vi "Read data manual.vi"() -> ()   [LabVIEW 2018]
uses:
  Controls/READ CAN CLUSTER.ctl
  Controls/CLUSTER.ctl
  CAN/Tacho/Conf/FGV States.ctl
  CAN/CAN Write Data/Application/Common VIs/Read File Data.ctl
  Controls/READ CAN DATA.ctl
  f1f4e13e-2694-4935-9f44-7f0de9cfde9a.vi
  56b8a145-6b6a-4ebf-8834-6d6c23b684ec.vi
panel:
  in  "Write":bool
  in  "WRITE DATA":T1[](array[typedef])
  in  "START WRITING":bool
  out "MESSAGES":string
  out "READ DATA":T1[](array[typedef])
  in  "stop":bool
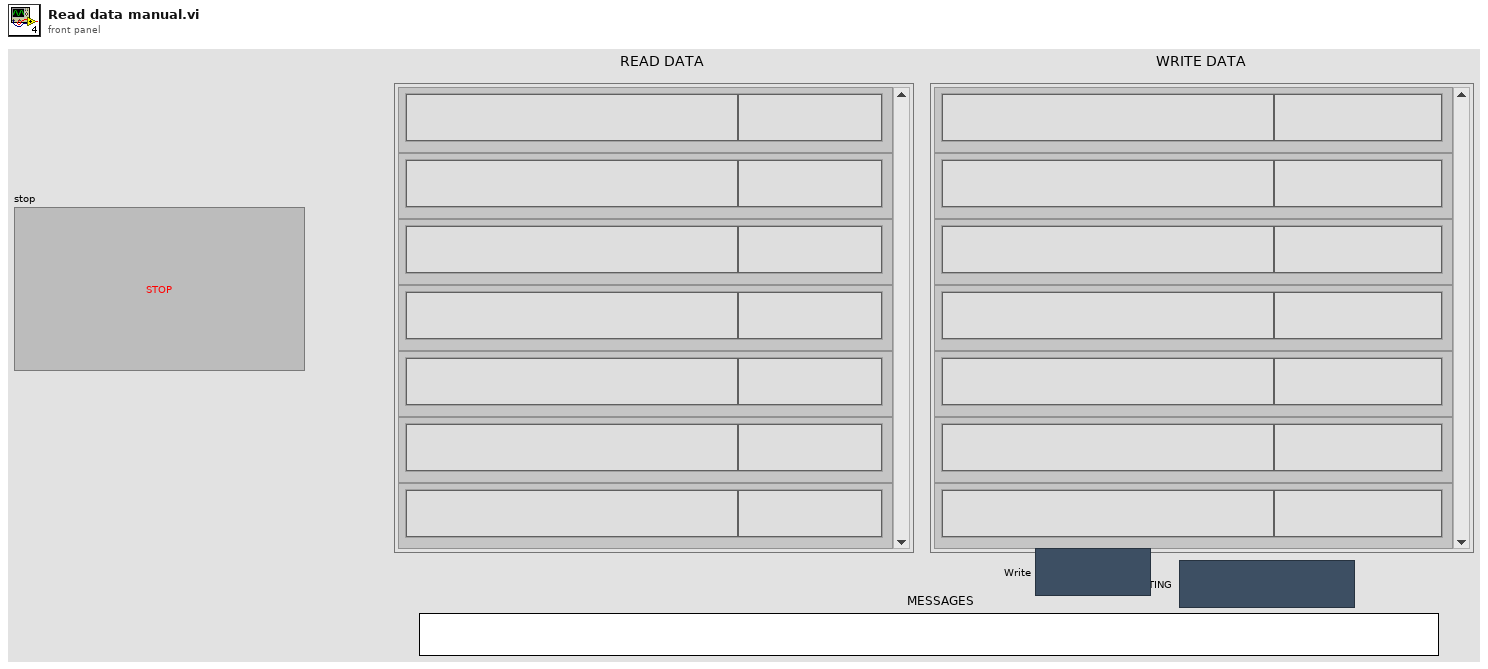
[diagram p1: front panel]
types:
  T1 = typedef "READ CAN CLUSTER.ctl" = cluster{"FUNCTION":string, "DATA":string}
  T2 = typedef "Read File Data.ctl" = enum16{"Get Data", "Set Data"}
  T3 = typedef "FGV States.ctl" = enum16{"OPEN", "READ", "CLOSE", "WRITE"}
  T4 = typedef "READ CAN DATA.ctl" = enum16{"SET", "GET"}
  T5 = typedef "CLUSTER.ctl" = cluster{"FUNCTION":string, "READ":bool, "WRITE":bool}
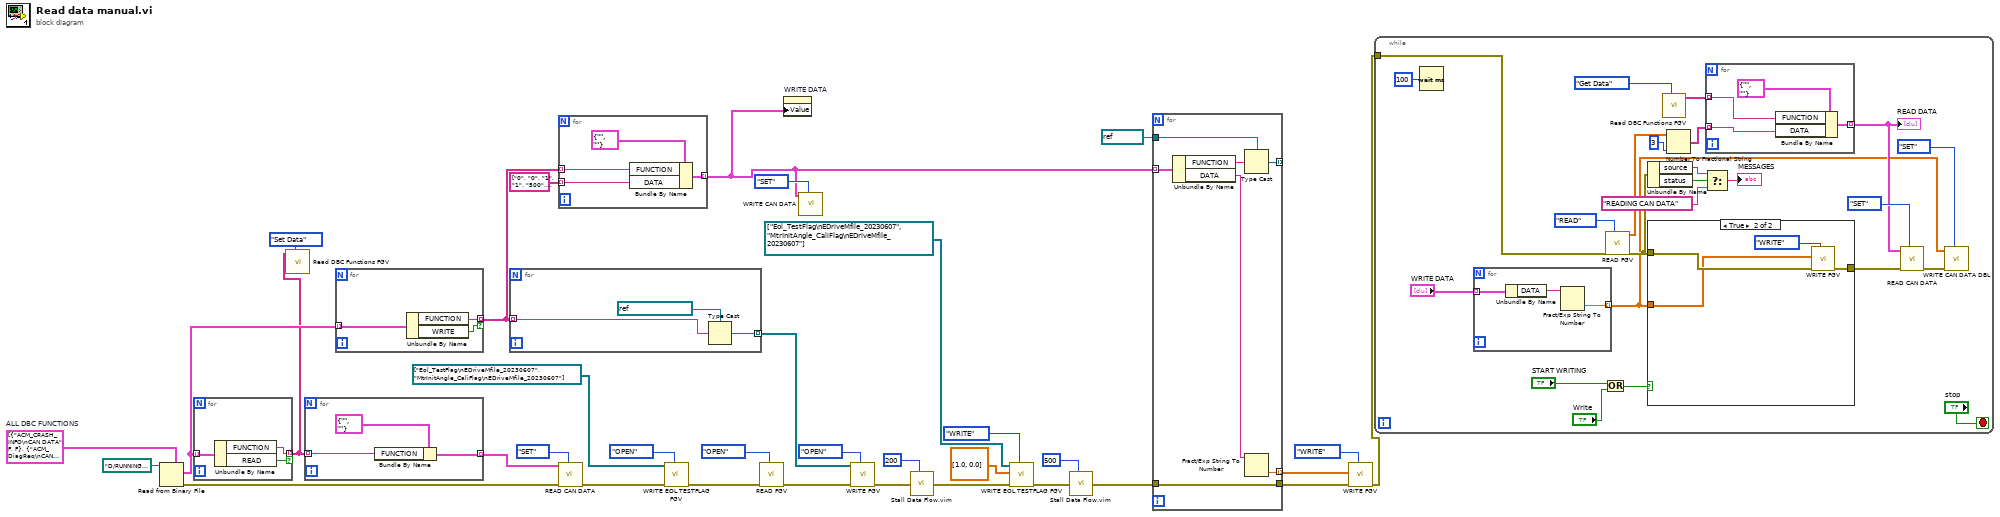
[diagram p0: block diagram]
diagram:
  w34 = T5[] [{"FUNCTION"="ACM_CRASH_INFO\nCAN DATA", "READ"=FALSE, "WRITE"=FALSE}, {"FUNCTION"="ACM_DiagReq\nCAN DATA", "READ"=FALSE, "WRITE"=FALSE}, {"FUNCTION"="ACM_DiagResp\nCAN DATA", "READ"=FALSE, "WRITE"=FALSE}, {"FUNCTION"="ACM_OCCUPANT_STATUS\nCAN DATA", "READ"=FALSE, "WRITE"=FALSE}, {"FUNCTION"="ACM_WarnMsg\nCAN DATA", "READ"=FALSE, "WRITE"=FALSE}, {"FUNCTION"="ADAS_AEB\nCAN DATA", "READ"=FALSE, "WRITE"=FALSE}, {"FUNCTION"="ADAS_AHB_DOW\nCAN DATA", "READ"=FALSE, "WRITE"=FALSE}, {"FUNCTION"="ADAS_APA_SLOT1INFO1\nCAN DATA", "READ"=FALSE, "WRITE"=FALSE}, {"FUNCTION"="ADAS_APA_SLOT1INFO2\nCAN DATA", "READ"=FALSE, "WRITE"=FALSE}, {"FUNCTION"="ADAS_APA_SLOT1INFO3\nCAN DATA", "READ"=FALSE, "WRITE"=FALSE}, {"FUNCTION"="ADAS_APA_SLOT2INFO1\nCAN DATA", "READ"=FALSE, "WRITE"=FALSE}, {"FUNCTION"="ADAS_APA_SLOT2INFO2\nCAN DATA", "READ"=FALSE, "WRITE"=FALSE}, {"FUNCTION"="ADAS_APA_SLOT2INFO3\nCAN DATA", "READ"=FALSE, "WRITE"=FALSE}, {"FUNCTION"="ADAS_APA_SLOT3INFO1\nCAN DATA", "READ"=FALSE, "WRITE"=FALSE}, {"FUNCTION"="ADAS_APA_SLOT3INFO2\nCAN DATA", "READ"=FALSE, "WRITE"=FALSE}, {"FUNCTION"="ADAS_APA_SLOT3INFO3\nCAN DATA", "READ"=FALSE, "WRITE"=FALSE}, {"FUNCTION"="ADAS_APA_SLOT4INFO1\nCAN DATA", "READ"=FALSE, "WRITE"=FALSE}, {"FUNCTION"="ADAS_APA_SLOT4INFO2\nCAN DATA", "READ"=FALSE, "WRITE"=FALSE}, {"FUNCTION"="ADAS_APA_SLOT4INFO3\nCAN DATA", "READ"=FALSE, "WRITE"=FALSE}, {"FUNCTION"="ADAS_APA_SLOT5INFO1\nCAN DATA", "READ"=FALSE, "WRITE"=FALSE}, {"FUNCTION"="ADAS_APA_SLOT5INFO2\nCAN DATA", "READ"=FALSE, "WRITE"=FALSE}, {"FUNCTION"="ADAS_APA_SLOT5INFO3\nCAN DATA", "READ"=FALSE, "WRITE"=FALSE}, {"FUNCTION"="ADAS_APA_SLOT6INFO1\nCAN DATA", "READ"=FALSE, "WRITE"=FALSE}, {"FUNCTION"="ADAS_APA_SLOT6INFO2\nCAN DATA", "READ"=FALSE, "WRITE"=FALSE}, {"FUNCTION"="ADAS_APA_SLOT6INFO3\nCAN DATA", "READ"=FALSE, "WRITE"=FALSE}, {"FUNCTION"="ADAS_AVM_Sts\nCAN DATA", "READ"=FALSE, "WRITE"=FALSE}, {"FUNCTION"="ADAS_BSD\nCAN DATA", "READ"=FALSE, "WRITE"=FALSE}, {"FUNCTION"="ADAS_CMP_ACC\nCAN DATA", "READ"=FALSE, "WRITE"=FALSE}, {"FUNCTION"="ADAS_CMP_CHECK\nCAN DATA", "READ"=FALSE, "WRITE"=FALSE}, {"FUNCTION"="ADAS_CMP_MHU\nCAN DATA", "READ"=FALSE, "WRITE"=FALSE}, {"FUNCTION"="ADAS_DMS_STATUS\nCAN DATA", "READ"=FALSE, "WRITE"=FALSE}, {"FUNCTION"="ADAS_DiagReq\nCAN DATA", "READ"=FALSE, "WRITE"=FALSE}, {"FUNCTION"="ADAS_DiagResp\nCAN DATA", "READ"=FALSE, "WRITE"=FALSE}, {"FUNCTION"="ADAS_ELK\nCAN DATA", "READ"=FALSE, "WRITE"=FALSE}, {"FUNCTION"="ADAS_FCW_RCTA\nCAN DATA", "READ"=FALSE, "WRITE"=FALSE}, {"FUNCTION"="ADAS_Immo_MHU\nCAN DATA", "READ"=FALSE, "WRITE"=FALSE}, {"FUNCTION"="ADAS_LDW_LKA\nCAN DATA", "READ"=FALSE, "WRITE"=FALSE}, {"FUNCTION"="ADAS_NM\nCAN DATA", "READ"=FALSE, "WRITE"=FALSE}, {"FUNCTION"="ADAS_PA\nCAN DATA", "READ"=FALSE, "WRITE"=FALSE}, {"FUNCTION"="ADAS_RP_Sts\nCAN DATA", "READ"=FALSE, "WRITE"=FALSE}, {"FUNCTION"="ADAS_Speed_Display\nCAN DATA", "READ"=FALSE, "WRITE"=FALSE}, {"FUNCTION"="ADAS_TSR_STATUS\nCAN DATA", "READ"=FALSE, "WRITE"=FALSE}, {"FUNCTION"="ADAS_WarnMsg\nCAN DATA", "READ"=FALSE, "WRITE"=FALSE}, {"FUNCTION"="AMP_DiagReq\nCAN DATA", "READ"=FALSE, "WRITE"=FALSE}, {"FUNCTION"="AMP_DiagResp\nCAN DATA", "READ"=FALSE, "WRITE"=FALSE}, {"FUNCTION"="AMP_MHUEQType\nCAN DATA", "READ"=FALSE, "WRITE"=FALSE}, {"FUNCTION"="AMP_MHU_Ann1_ModeSET\nCAN DATA", "READ"=FALSE, "WRITE"=FALSE}, {"FUNCTION"="AMP_MHU_Ann1_PromptsSET\nCAN DATA", "READ"=FALSE, "WRITE"=FALSE}, {"FUNCTION"="AMP_MHU_Ann2_SpeakerSET\nCAN DATA", "READ"=FALSE, "WRITE"=FALSE}, {"FUNCTION"="AMP_MHU_SET\nCAN DATA", "READ"=FALSE, "WRITE"=FALSE}, {"FUNCTION"="AMP_NM\nCAN DATA", "READ"=FALSE, "WRITE"=FALSE}, {"FUNCTION"="AMP_rDiagReq\nCAN DATA", "READ"=FALSE, "WRITE"=FALSE}, {"FUNCTION"="AMP_rDiagResp\nCAN DATA", "READ"=FALSE, "WRITE"=FALSE}, {"FUNCTION"="APA_FEEDBACK_MHU\nCAN DATA", "READ"=FALSE, "WRITE"=FALSE}, {"FUNCTION"="APA_SENSOR\nCAN DATA", "READ"=FALSE, "WRITE"=FALSE}, {"FUNCTION"="APM_DiagReq\nCAN DATA", "READ"=FALSE, "WRITE"=FALSE}, {"FUNCTION"="APM_DiagResp\nCAN DATA", "READ"=FALSE, "WRITE"=FALSE}, {"FUNCTION"="APM_WINDOW_POS\nCAN DATA", "READ"=FALSE, "WRITE"=FALSE}, {"FUNCTION"="APM_WarnMsg\nCAN DATA", "READ"=FALSE, "WRITE"=FALSE}, {"FUNCTION"="ASU_DiagReq\nCAN DATA", "READ"=FALSE, "WRITE"=FALSE}, {"FUNCTION"="ASU_DiagResp\nCAN DATA", "READ"=FALSE, "WRITE"=FALSE}, {"FUNCTION"="AVAS_DiagReq\nCAN DATA", "READ"=FALSE, "WRITE"=FALSE}, {"FUNCTION"="AVAS_DiagResp\nCAN DATA", "READ"=FALSE, "WRITE"=FALSE}, {"FUNCTION"="AVAS_STATUS\nCAN DATA", "READ"=FALSE, "WRITE"=FALSE}, {"FUNCTION"="BCM_ALM_warning\nCAN DATA", "READ"=FALSE, "WRITE"=FALSE}, {"FUNCTION"="BCM_BPM_DiagReq\nCAN DATA", "READ"=FALSE, "WRITE"=FALSE}, {"FUNCTION"="BCM_BPM_DiagResp\nCAN DATA", "READ"=FALSE, "WRITE"=FALSE}, {"FUNCTION"="BCM_CLAMP_STAT\nCAN DATA", "READ"=FALSE, "WRITE"=FALSE}, {"FUNCTION"="BCM_Comfort_Confirm_sts\nCAN DATA", "READ"=FALSE, "WRITE"=FALSE}, {"FUNCTION"="BCM_DiagReq\nCAN DATA", "READ"=FALSE, "WRITE"=FALSE}, {"FUNCTION"="BCM_DiagResp\nCAN DATA", "READ"=FALSE, "WRITE"=FALSE}, {"FUNCTION"="BCM_ENERGY_MANAGEMENT\nCAN DATA", "READ"=FALSE, "WRITE"=FALSE}, {"FUNCTION"="BCM_ENTRY_CONTROL\nCAN DATA", "READ"=FALSE, "WRITE"=FALSE}, {"FUNCTION"="BCM_FKS_STATUS\nCAN DATA", "READ"=FALSE, "WRITE"=FALSE}, {"FUNCTION"="BCM_LIGHT\nCAN DATA", "READ"=FALSE, "WRITE"=FALSE}, {"FUNCTION"="BCM_LOGICAL_CLAMP\nCAN DATA", "READ"=FALSE, "WRITE"=FALSE}, {"FUNCTION"="BCM_Mirror_Confirm_sts\nCAN DATA", "READ"=FALSE, "WRITE"=FALSE}, {"FUNCTION"="BCM_ODO\nCAN DATA", "READ"=FALSE, "WRITE"=FALSE}, {"FUNCTION"="BCM_RainLightSnr\nCAN DATA", "READ"=FALSE, "WRITE"=FALSE}, {"FUNCTION"="BCM_SCM_LIN_Info\nCAN DATA", "READ"=FALSE, "WRITE"=FALSE}, {"FUNCTION"="BCM_STAT_CENTRAL_LOCK\nCAN DATA", "READ"=FALSE, "WRITE"=FALSE}, {"FUNCTION"="BCM_STAT_DOOR_FLAP\nCAN DATA", "READ"=FALSE, "WRITE"=FALSE}, {"FUNCTION"="BCM_SunroofSts\nCAN DATA", "READ"=FALSE, "WRITE"=FALSE}, {"FUNCTION"="BCM_SunshadeSts\nCAN DATA", "READ"=FALSE, "WRITE"=FALSE}, {"FUNCTION"="BCM_SwitchSts\nCAN DATA", "READ"=FALSE, "WRITE"=FALSE}, {"FUNCTION"="BCM_TERMINAL\nCAN DATA", "READ"=FALSE, "WRITE"=FALSE}, {"FUNCTION"="BCM_VEHICLE_IDENT_NUMBER\nCAN DATA", "READ"=FALSE, "WRITE"=FALSE}, {"FUNCTION"="BCM_VOLTAGE\nCAN DATA", "READ"=FALSE, "WRITE"=FALSE}, {"FUNCTION"="BCM_WarnMsg\nCAN DATA", "READ"=FALSE, "WRITE"=FALSE}, {"FUNCTION"="BMS_CellTemp\nCAN DATA", "READ"=FALSE, "WRITE"=FALSE}, {"FUNCTION"="BMS_ChgParamReq\nCAN DATA", "READ"=FALSE, "WRITE"=FALSE}, {"FUNCTION"="BMS_CurMeas\nCAN DATA", "READ"=FALSE, "WRITE"=FALSE}, {"FUNCTION"="BMS_DiagReq\nCAN DATA", "READ"=FALSE, "WRITE"=FALSE}, {"FUNCTION"="BMS_DiagResp\nCAN DATA", "READ"=FALSE, "WRITE"=FALSE}, {"FUNCTION"="BMS_HVMeas1\nCAN DATA", "READ"=FALSE, "WRITE"=FALSE}, {"FUNCTION"="BMS_Sts\nCAN DATA", "READ"=FALSE, "WRITE"=FALSE}, {"FUNCTION"="BMS_WarnMsg\nCAN DATA", "READ"=FALSE, "WRITE"=FALSE}, {"FUNCTION"="CCUF_DiagReq\nCAN DATA", "READ"=FALSE, "WRITE"=FALSE}, {"FUNCTION"="CCUF_DiagResp\nCAN DATA", "READ"=FALSE, "WRITE"=FALSE}, {"FUNCTION"="CCUR_DiagReq\nCAN DATA", "READ"=FALSE, "WRITE"=FALSE}, {"FUNCTION"="CCUR_DiagResp\nCAN DATA", "READ"=FALSE, "WRITE"=FALSE}, {"FUNCTION"="CCU_STATUS\nCAN DATA", "READ"=FALSE, "WRITE"=FALSE}, {"FUNCTION"="CCU_TEMP_PRESSURE\nCAN DATA", "READ"=FALSE, "WRITE"=FALSE}, {"FUNCTION"="CCU_WarnMsg\nCAN DATA", "READ"=FALSE, "WRITE"=FALSE}, {"FUNCTION"="CPD_DiagReq\nCAN DATA", "READ"=FALSE, "WRITE"=FALSE}, {"FUNCTION"="CPD_DiagResp\nCAN DATA", "READ"=FALSE, "WRITE"=FALSE}, {"FUNCTION"="CPD_NM\nCAN DATA", "READ"=FALSE, "WRITE"=FALSE}, {"FUNCTION"="CPD_OUTPUT\nCAN DATA", "READ"=FALSE, "WRITE"=FALSE}, {"FUNCTION"="CPD_WarnMsg\nCAN DATA", "READ"=FALSE, "WRITE"=FALSE}, {"FUNCTION"="CPD_rDiagReq\nCAN DATA", "READ"=FALSE, "WRITE"=FALSE}, {"FUNCTION"="CPD_rDiagResp\nCAN DATA", "READ"=FALSE, "WRITE"=FALSE}, {"FUNCTION"="Camera_Lane\nCAN DATA", "READ"=FALSE, "WRITE"=FALSE}, {"FUNCTION"="Camera_Object01\nCAN DATA", "READ"=FALSE, "WRITE"=FALSE}, {"FUNCTION"="Camera_Object02\nCAN DATA", "READ"=FALSE, "WRITE"=FALSE}, {"FUNCTION"="Camera_Object03\nCAN DATA", "READ"=FALSE, "WRITE"=FALSE}, {"FUNCTION"="Camera_Object04\nCAN DATA", "READ"=FALSE, "WRITE"=FALSE}, {"FUNCTION"="Camera_Object05\nCAN DATA", "READ"=FALSE, "WRITE"=FALSE}, {"FUNCTION"="Camera_Object06\nCAN DATA", "READ"=FALSE, "WRITE"=FALSE}, {"FUNCTION"="Camera_leftlane\nCAN DATA", "READ"=FALSE, "WRITE"=FALSE}, {"FUNCTION"="Camera_rightlane\nCAN DATA", "READ"=FALSE, "WRITE"=FALSE}, {"FUNCTION"="DCM_APM_DiagReq\nCAN DATA", "READ"=FALSE, "WRITE"=FALSE}, {"FUNCTION"="DCM_APM_DiagResp\nCAN DATA", "READ"=FALSE, "WRITE"=FALSE}, {"FUNCTION"="DIAG_Req_All_CAN\nCAN DATA", "READ"=FALSE, "WRITE"=FALSE}, {"FUNCTION"="DIAG_Req_All_Ecu\nCAN DATA", "READ"=FALSE, "WRITE"=FALSE}, {"FUNCTION"="DIAG_Req_Info\nCAN DATA", "READ"=FALSE, "WRITE"=FALSE}, {"FUNCTION"="DMS_Status\nCAN DATA", "READ"=FALSE, "WRITE"=FALSE}, {"FUNCTION"="Diag_Request_ECU\nCAN DATA", "READ"=FALSE, "WRITE"=FALSE}, {"FUNCTION"="EASC_Confirm_sts\nCAN DATA", "READ"=FALSE, "WRITE"=FALSE}, {"FUNCTION"="EASC_DiagReq\nCAN DATA", "READ"=FALSE, "WRITE"=FALSE}, {"FUNCTION"="EASC_DiagResp\nCAN DATA", "READ"=FALSE, "WRITE"=FALSE}, {"FUNCTION"="EASC_NM\nCAN DATA", "READ"=FALSE, "WRITE"=FALSE}, {"FUNCTION"="EASC_WarnMsg\nCAN DATA", "READ"=FALSE, "WRITE"=FALSE}, {"FUNCTION"="EASC_rDiagReq\nCAN DATA", "READ"=FALSE, "WRITE"=FALSE}, {"FUNCTION"="EASC_rDiagResp\nCAN DATA", "READ"=FALSE, "WRITE"=FALSE}, {"FUNCTION"="EDS_F_DiagReq\nCAN DATA", "READ"=FALSE, "WRITE"=FALSE}, {"FUNCTION"="EDS_F_DiagResp\nCAN DATA", "READ"=FALSE, "WRITE"=FALSE}, {"FUNCTION"="EDS_F_WarnMsg\nCAN DATA", "READ"=FALSE, "WRITE"=FALSE}, {"FUNCTION"="EDS_OutPut_FR\nCAN DATA", "READ"=FALSE, "WRITE"=FALSE}, {"FUNCTION"="EDS_OutPut_RR\nCAN DATA", "READ"=FALSE, "WRITE"=FALSE}, {"FUNCTION"="EDS_R_DiagReq\nCAN DATA", "READ"=FALSE, "WRITE"=FALSE}, {"FUNCTION"="EDS_R_DiagResp\nCAN DATA", "READ"=FALSE, "WRITE"=FALSE}, {"FUNCTION"="EDS_R_WarnMsg\nCAN DATA", "READ"=FALSE, "WRITE"=FALSE}, {"FUNCTION"="EPS2_DiagReq\nCAN DATA", "READ"=FALSE, "WRITE"=FALSE}, {"FUNCTION"="EPS2_DiagResp\nCAN DATA", "READ"=FALSE, "WRITE"=FALSE}, {"FUNCTION"="EPS_DiagReq\nCAN DATA", "READ"=FALSE, "WRITE"=FALSE}, {"FUNCTION"="EPS_DiagResp\nCAN DATA", "READ"=FALSE, "WRITE"=FALSE}, {"FUNCTION"="EPS_WarnMsg\nCAN DATA", "READ"=FALSE, "WRITE"=FALSE}, {"FUNCTION"="ETG_DiagReq\nCAN DATA", "READ"=FALSE, "WRITE"=FALSE}, {"FUNCTION"="ETG_DiagResp\nCAN DATA", "READ"=FALSE, "WRITE"=FALSE}, {"FUNCTION"="ETG_STATUS\nCAN DATA", "READ"=FALSE, "WRITE"=FALSE}, {"FUNCTION"="ETG_WarnMsg\nCAN DATA", "READ"=FALSE, "WRITE"=FALSE}, {"FUNCTION"="GS_DiagReq\nCAN DATA", "READ"=FALSE, "WRITE"=FALSE}, {"FUNCTION"="GS_DiagResp\nCAN DATA", "READ"=FALSE, "WRITE"=FALSE}, {"FUNCTION"="GS_WarnMsg\nCAN DATA", "READ"=FALSE, "WRITE"=FALSE}, {"FUNCTION"="GW_BCM_Immo_MHU_Byte\nCAN DATA", "READ"=FALSE, "WRITE"=FALSE}, {"FUNCTION"="GW_BCM_RemoteCtrlSts\nCAN DATA", "READ"=FALSE, "WRITE"=FALSE}, {"FUNCTION"="HOD_Heating\nCAN DATA", "READ"=FALSE, "WRITE"=FALSE}, {"FUNCTION"="HOD_Heating_FDBK\nCAN DATA", "READ"=FALSE, "WRITE"=FALSE}, {"FUNCTION"="HUD_DiagReq\nCAN DATA", "READ"=FALSE, "WRITE"=FALSE}, {"FUNCTION"="HUD_DiagResp\nCAN DATA", "READ"=FALSE, "WRITE"=FALSE}, {"FUNCTION"="HUD_ECU_Status\nCAN DATA", "READ"=FALSE, "WRITE"=FALSE}, {"FUNCTION"="HUD_NM\nCAN DATA", "READ"=FALSE, "WRITE"=FALSE}, {"FUNCTION"="HUD_State\nCAN DATA", "READ"=FALSE, "WRITE"=FALSE}, {"FUNCTION"="HUD_WarnMsg\nCAN DATA", "READ"=FALSE, "WRITE"=FALSE}, {"FUNCTION"="HUD_rDiagReq\nCAN DATA", "READ"=FALSE, "WRITE"=FALSE}, {"FUNCTION"="HUD_rDiagResp\nCAN DATA", "READ"=FALSE, "WRITE"=FALSE}, {"FUNCTION"="IC_BORD_COMP_TRIP_A\nCAN DATA", "READ"=FALSE, "WRITE"=FALSE}, {"FUNCTION"="IC_BORD_COMP_TRIP_Auto\nCAN DATA", "READ"=FALSE, "WRITE"=FALSE}, {"FUNCTION"="IC_BORD_COMP_TRIP_B\nCAN DATA", "READ"=FALSE, "WRITE"=FALSE}, {"FUNCTION"="IC_MILEAGE\nCAN DATA", "READ"=FALSE, "WRITE"=FALSE}, {"FUNCTION"="IC_ODO\nCAN DATA", "READ"=FALSE, "WRITE"=FALSE}, {"FUNCTION"="IC_RELATIVIME\nCAN DATA", "READ"=FALSE, "WRITE"=FALSE}, {"FUNCTION"="IC_SENSOR\nCAN DATA", "READ"=FALSE, "WRITE"=FALSE}, {"FUNCTION"="IC_STAT_AIRBAG\nCAN DATA", "READ"=FALSE, "WRITE"=FALSE}, {"FUNCTION"="IDB_ACC_LONG_LAT_YAW\nCAN DATA", "READ"=FALSE, "WRITE"=FALSE}, {"FUNCTION"="IDB_DiagReq\nCAN DATA", "READ"=FALSE, "WRITE"=FALSE}, {"FUNCTION"="IDB_DiagResp\nCAN DATA", "READ"=FALSE, "WRITE"=FALSE}, {"FUNCTION"="IDB_EPB_STATUS\nCAN DATA", "READ"=FALSE, "WRITE"=FALSE}, {"FUNCTION"="IDB_FUNCTION\nCAN DATA", "READ"=FALSE, "WRITE"=FALSE}, {"FUNCTION"="IDB_MILEAGE\nCAN DATA", "READ"=FALSE, "WRITE"=FALSE}, {"FUNCTION"="IDB_STATUS\nCAN DATA", "READ"=FALSE, "WRITE"=FALSE}, {"FUNCTION"="IDB_V_VEH\nCAN DATA", "READ"=FALSE, "WRITE"=FALSE}, {"FUNCTION"="IDB_WarnMsg\nCAN DATA", "READ"=FALSE, "WRITE"=FALSE}, {"FUNCTION"="LDML_LIGHT\nCAN DATA", "READ"=FALSE, "WRITE"=FALSE}, {"FUNCTION"="LDMR_LIGHT\nCAN DATA", "READ"=FALSE, "WRITE"=FALSE}, {"FUNCTION"="LDM_L_DiagReq\nCAN DATA", "READ"=FALSE, "WRITE"=FALSE}, {"FUNCTION"="LDM_L_DiagResp\nCAN DATA", "READ"=FALSE, "WRITE"=FALSE}, {"FUNCTION"="LDM_R_DiagReq\nCAN DATA", "READ"=FALSE, "WRITE"=FALSE}, {"FUNCTION"="LDM_R_DiagResp\nCAN DATA", "READ"=FALSE, "WRITE"=FALSE}, {"FUNCTION"="MFS_Control_Button\nCAN DATA", "READ"=FALSE, "WRITE"=FALSE}, {"FUNCTION"="MHU_ADAS_RP_Ctrl\nCAN DATA", "READ"=FALSE, "WRITE"=FALSE}, {"FUNCTION"="MHU_ADAS_RSSI\nCAN DATA", "READ"=FALSE, "WRITE"=FALSE}, {"FUNCTION"="MHU_ADAS_req\nCAN DATA", "READ"=FALSE, "WRITE"=FALSE}, {"FUNCTION"="MHU_AMP_Ann1_ModeSET\nCAN DATA", "READ"=FALSE, "WRITE"=FALSE}, {"FUNCTION"="MHU_AMP_Ann1_PromptsSET\nCAN DATA", "READ"=FALSE, "WRITE"=FALSE}, {"FUNCTION"="MHU_AMP_Ann2_SpeakerSET\nCAN DATA", "READ"=FALSE, "WRITE"=FALSE}, {"FUNCTION"="MHU_AmpEQType\nCAN DATA", "READ"=FALSE, "WRITE"=FALSE}, {"FUNCTION"="MHU_AmpSET\nCAN DATA", "READ"=FALSE, "WRITE"=FALSE}, {"FUNCTION"="MHU_Auth_Immo\nCAN DATA", "READ"=FALSE, "WRITE"=FALSE}, {"FUNCTION"="MHU_Auth_Immo_ADAS\nCAN DATA", "READ"=FALSE, "WRITE"=FALSE}, {"FUNCTION"="MHU_Avas_Setting\nCAN DATA", "READ"=FALSE, "WRITE"=FALSE}, {"FUNCTION"="MHU_BCM_Color_Req\nCAN DATA", "READ"=FALSE, "WRITE"=FALSE}, {"FUNCTION"="MHU_BCM_DoorsCtrl\nCAN DATA", "READ"=FALSE, "WRITE"=FALSE}, {"FUNCTION"="MHU_BCM_HornLightControl\nCAN DATA", "READ"=FALSE, "WRITE"=FALSE}, {"FUNCTION"="MHU_BCM_IntensityTiming_Req\nCAN DATA", "READ"=FALSE, "WRITE"=FALSE}, {"FUNCTION"="MHU_BCM_RemoteClampCtrl\nCAN DATA", "READ"=FALSE, "WRITE"=FALSE}, {"FUNCTION"="MHU_CCUF_ClimateSetting\nCAN DATA", "READ"=FALSE, "WRITE"=FALSE}, {"FUNCTION"="MHU_CCUR_ClimateSetting\nCAN DATA", "READ"=FALSE, "WRITE"=FALSE}, {"FUNCTION"="MHU_CPD_Confirm\nCAN DATA", "READ"=FALSE, "WRITE"=FALSE}, {"FUNCTION"="MHU_CarMode_Switch\nCAN DATA", "READ"=FALSE, "WRITE"=FALSE}, {"FUNCTION"="MHU_ComfortSetting\nCAN DATA", "READ"=FALSE, "WRITE"=FALSE}, {"FUNCTION"="MHU_DATE_TIME\nCAN DATA", "READ"=FALSE, "WRITE"=FALSE}, {"FUNCTION"="MHU_DIGIT_SPEED\nCAN DATA", "READ"=FALSE, "WRITE"=FALSE}, {"FUNCTION"="MHU_DMS_STATUS\nCAN DATA", "READ"=FALSE, "WRITE"=FALSE}, {"FUNCTION"="MHU_DRIVER_INFO\nCAN DATA", "READ"=FALSE, "WRITE"=FALSE}, {"FUNCTION"="MHU_DiagReq\nCAN DATA", "READ"=FALSE, "WRITE"=FALSE}, {"FUNCTION"="MHU_DiagResp\nCAN DATA", "READ"=FALSE, "WRITE"=FALSE}, {"FUNCTION"="MHU_DoorSetting\nCAN DATA", "READ"=FALSE, "WRITE"=FALSE}, {"FUNCTION"="MHU_EvSetting\nCAN DATA", "READ"=FALSE, "WRITE"=FALSE}, {"FUNCTION"="MHU_FEEDBACK_APA\nCAN DATA", "READ"=FALSE, "WRITE"=FALSE}, {"FUNCTION"="MHU_FOTA_ReqAll\nCAN DATA", "READ"=FALSE, "WRITE"=FALSE}, {"FUNCTION"="MHU_FOTA_STATUS\nCAN DATA", "READ"=FALSE, "WRITE"=FALSE}, {"FUNCTION"="MHU_HEADLAMP_CTL\nCAN DATA", "READ"=FALSE, "WRITE"=FALSE}, {"FUNCTION"="MHU_HUD_BASE\nCAN DATA", "READ"=FALSE, "WRITE"=FALSE}, {"FUNCTION"="MHU_HUD_Info_1\nCAN DATA", "READ"=FALSE, "WRITE"=FALSE}, {"FUNCTION"="MHU_HUD_NAV_DISP\nCAN DATA", "READ"=FALSE, "WRITE"=FALSE}, {"FUNCTION"="MHU_HUD_NAV_GuidanceCont\nCAN DATA", "READ"=FALSE, "WRITE"=FALSE}, {"FUNCTION"="MHU_HudPositionSetting\nCAN DATA", "READ"=FALSE, "WRITE"=FALSE}, {"FUNCTION"="MHU_HudSetting\nCAN DATA", "READ"=FALSE, "WRITE"=FALSE}, {"FUNCTION"="MHU_IDB_Mode_Select\nCAN DATA", "READ"=FALSE, "WRITE"=FALSE}, {"FUNCTION"="MHU_ISA_Speed\nCAN DATA", "READ"=FALSE, "WRITE"=FALSE}, {"FUNCTION"="MHU_LightSetting\nCAN DATA", "READ"=FALSE, "WRITE"=FALSE}, {"FUNCTION"="MHU_MirrorAdjust\nCAN DATA", "READ"=FALSE, "WRITE"=FALSE}, {"FUNCTION"="MHU_NAV_JUNC_INFO\nCAN DATA", "READ"=FALSE, "WRITE"=FALSE}, {"FUNCTION"="MHU_NM\nCAN DATA", "READ"=FALSE, "WRITE"=FALSE}, {"FUNCTION"="MHU_SEAT_CONTROL\nCAN DATA", "READ"=FALSE, "WRITE"=FALSE}, {"FUNCTION"="MHU_STATUS\nCAN DATA", "READ"=FALSE, "WRITE"=FALSE}, {"FUNCTION"="MHU_SeatVentHeat\nCAN DATA", "READ"=FALSE, "WRITE"=FALSE}, {"FUNCTION"="MHU_SteeringAdjust\nCAN DATA", "READ"=FALSE, "WRITE"=FALSE}, {"FUNCTION"="MHU_UserProfile\nCAN DATA", "READ"=FALSE, "WRITE"=FALSE}, {"FUNCTION"="MHU_WindowSetting\nCAN DATA", "READ"=FALSE, "WRITE"=FALSE}, {"FUNCTION"="MRGEN_DiagReq\nCAN DATA", "READ"=FALSE, "WRITE"=FALSE}, {"FUNCTION"="MRGEN_DiagResp\nCAN DATA", "READ"=FALSE, "WRITE"=FALSE}, {"FUNCTION"="OCS_P_DiagReq\nCAN DATA", "READ"=FALSE, "WRITE"=FALSE}, {"FUNCTION"="OCS_P_DiagResp\nCAN DATA", "READ"=FALSE, "WRITE"=FALSE}, {"FUNCTION"="POD_DCDC_DiagReq\nCAN DATA", "READ"=FALSE, "WRITE"=FALSE}, {"FUNCTION"="POD_DCDC_DiagResp\nCAN DATA", "READ"=FALSE, "WRITE"=FALSE}, {"FUNCTION"="POD_GW_Request\nCAN DATA", "READ"=FALSE, "WRITE"=FALSE}, {"FUNCTION"="POD_GW_Response\nCAN DATA", "READ"=FALSE, "WRITE"=FALSE}, {"FUNCTION"="POD_OBC_DiagReq\nCAN DATA", "READ"=FALSE, "WRITE"=FALSE}, {"FUNCTION"="POD_OBC_DiagResp\nCAN DATA", "READ"=FALSE, "WRITE"=FALSE}, {"FUNCTION"="POD_WarnMsg\nCAN DATA", "READ"=FALSE, "WRITE"=FALSE}, {"FUNCTION"="PSM_D_DiagReq\nCAN DATA", "READ"=FALSE, "WRITE"=FALSE}, {"FUNCTION"="PSM_D_DiagResp\nCAN DATA", "READ"=FALSE, "WRITE"=FALSE}, {"FUNCTION"="PSM_D_SEAT_CONTROL\nCAN DATA", "READ"=FALSE, "WRITE"=FALSE}, {"FUNCTION"="PSM_SEAT_POSITION\nCAN DATA", "READ"=FALSE, "WRITE"=FALSE}, {"FUNCTION"="PSM_WarnMsg\nCAN DATA", "READ"=FALSE, "WRITE"=FALSE}, {"FUNCTION"="RCU_DiagReq\nCAN DATA", "READ"=FALSE, "WRITE"=FALSE}, {"FUNCTION"="RCU_DiagResp\nCAN DATA", "READ"=FALSE, "WRITE"=FALSE}, {"FUNCTION"="RCU_WarnMsg\nCAN DATA", "READ"=FALSE, "WRITE"=FALSE}, {"FUNCTION"="SAS_Sensor\nCAN DATA", "READ"=FALSE, "WRITE"=FALSE}, {"FUNCTION"="SCAM_DiagReq\nCAN DATA", "READ"=FALSE, "WRITE"=FALSE}, {"FUNCTION"="SCAM_DiagResp\nCAN DATA", "READ"=FALSE, "WRITE"=FALSE}, {"FUNCTION"="SCM_Raw_Status\nCAN DATA", "READ"=FALSE, "WRITE"=FALSE}, {"FUNCTION"="SHVU_F_Confirm_Sts\nCAN DATA", "READ"=FALSE, "WRITE"=FALSE}, {"FUNCTION"="SHVU_F_DiagReq\nCAN DATA", "READ"=FALSE, "WRITE"=FALSE}, {"FUNCTION"="SHVU_F_DiagResp\nCAN DATA", "READ"=FALSE, "WRITE"=FALSE}, {"FUNCTION"="SHVU_R_Confirm_Sts\nCAN DATA", "READ"=FALSE, "WRITE"=FALSE}, {"FUNCTION"="SHVU_R_DiagReq\nCAN DATA", "READ"=FALSE, "WRITE"=FALSE}, {"FUNCTION"="SHVU_R_DiagResp\nCAN DATA", "READ"=FALSE, "WRITE"=FALSE}, {"FUNCTION"="SRR_FL_DiagReq\nCAN DATA", "READ"=FALSE, "WRITE"=FALSE}, {"FUNCTION"="SRR_FL_DiagResp\nCAN DATA", "READ"=FALSE, "WRITE"=FALSE}, {"FUNCTION"="SRR_FR_DiagReq\nCAN DATA", "READ"=FALSE, "WRITE"=FALSE}, {"FUNCTION"="SRR_FR_DiagResp\nCAN DATA", "READ"=FALSE, "WRITE"=FALSE}, {"FUNCTION"="SRR_RL_DiagReq\nCAN DATA", "READ"=FALSE, "WRITE"=FALSE}, {"FUNCTION"="SRR_RL_DiagResp\nCAN DATA", "READ"=FALSE, "WRITE"=FALSE}, {"FUNCTION"="SRR_RR_DiagReq\nCAN DATA", "READ"=FALSE, "WRITE"=FALSE}, {"FUNCTION"="SRR_RR_DiagResp\nCAN DATA", "READ"=FALSE, "WRITE"=FALSE}, {"FUNCTION"="SeatMassage_Input\nCAN DATA", "READ"=FALSE, "WRITE"=FALSE}, {"FUNCTION"="SeatMassage_Output\nCAN DATA", "READ"=FALSE, "WRITE"=FALSE}, {"FUNCTION"="Sensor_Fault\nCAN DATA", "READ"=FALSE, "WRITE"=FALSE}, {"FUNCTION"="TPMS_TirePressure\nCAN DATA", "READ"=FALSE, "WRITE"=FALSE}, {"FUNCTION"="TRM_DiagReq\nCAN DATA", "READ"=FALSE, "WRITE"=FALSE}, {"FUNCTION"="TRM_DiagResp\nCAN DATA", "READ"=FALSE, "WRITE"=FALSE}, {"FUNCTION"="TRM_WarnMsg\nCAN DATA", "READ"=FALSE, "WRITE"=FALSE}, {"FUNCTION"="VCU_ChargingConnection\nCAN DATA", "READ"=FALSE, "WRITE"=FALSE}, {"FUNCTION"="VCU_DiagReq\nCAN DATA", "READ"=FALSE, "WRITE"=FALSE}, {"FUNCTION"="VCU_DiagResp\nCAN DATA", "READ"=FALSE, "WRITE"=FALSE}, {"FUNCTION"="VCU_HMI_Info\nCAN DATA", "READ"=FALSE, "WRITE"=FALSE}, {"FUNCTION"="VCU_HV_DrvSys_status\nCAN DATA", "READ"=FALSE, "WRITE"=FALSE}, {"FUNCTION"="VCU_HVsystem_status\nCAN DATA", "READ"=FALSE, "WRITE"=FALSE}, {"FUNCTION"="VCU_MHU_info\nCAN DATA", "READ"=FALSE, "WRITE"=FALSE}, {"FUNCTION"="VCU_WarnMsg\nCAN DATA", "READ"=FALSE, "WRITE"=FALSE}, {"FUNCTION"="WLC_Status\nCAN DATA", "READ"=FALSE, "WRITE"=FALSE}, {"FUNCTION"="WLC_Status_2\nCAN DATA", "READ"=FALSE, "WRITE"=FALSE}, {"FUNCTION"="XGW_DiagReq\nCAN DATA", "READ"=FALSE, "WRITE"=FALSE}, {"FUNCTION"="XGW_DiagResp\nCAN DATA", "READ"=FALSE, "WRITE"=FALSE}, {"FUNCTION"="XGW_FOTA_StsConfirm\nCAN DATA", "READ"=FALSE, "WRITE"=FALSE}, {"FUNCTION"="XGW_HCMInfo\nCAN DATA", "READ"=FALSE, "WRITE"=FALSE}, {"FUNCTION"="XGW_Info_Collect\nCAN DATA", "READ"=FALSE, "WRITE"=FALSE}, {"FUNCTION"="XGW_NM\nCAN DATA", "READ"=FALSE, "WRITE"=FALSE}, {"FUNCTION"="XGW_System_Info\nCAN DATA", "READ"=FALSE, "WRITE"=FALSE}, {"FUNCTION"="XGW_WarnMsg\nCAN DATA", "READ"=FALSE, "WRITE"=FALSE}, {"FUNCTION"="YSS_DiagReq\nCAN DATA", "READ"=FALSE, "WRITE"=FALSE}, {"FUNCTION"="YSS_DiagResp\nCAN DATA", "READ"=FALSE, "WRITE"=FALSE}]  # ALL DBC FUNCTIONS
  n1 = Read from Binary File(5:w34, 11:path "D:/RUNNING PROJECT/FEV/#0253/9. Softcode/Source Code/Data/Models/TACO/ALL DBC.txt" ("file (use dialog)")) -> (0:w5:errorcluster, 2:w33:T5[])  [unwired: 4 in, 2 out]
  n2 = for {
    tunnel: w33 -> [w37] mode=indexing
    tunnel: [w36] -> w1 mode=indexing if=w35
    n3 = Unbundle By Name(w37) -> ("FUNCTION"=w36:string, "READ"=w35:bool)
  }
  n4 = call "Read DBC Functions FGV.vi"("Enum"=Read_File_Data."Set Data", "DBC FUNCTIONS IN"=w1) -> ()  [unwired: 8 in, 2 out]
  n5 = for {
    tunnel: w1 -> [w39] mode=indexing
    tunnel: [w38] -> w30 mode=indexing
    n6 = Bundle By Name(cluster=T1 {"FUNCTION"="", "DATA"=""} ("FUNCTIONS"), "FUNCTION"=w39) -> (w38:T1)
  }
  n7 = for {
    tunnel: w33 -> [w43] mode=indexing
    tunnel: [w42] -> w8 mode=indexing if=w41
    n8 = Unbundle By Name(w43) -> ("FUNCTION"=w42:string, "WRITE"=w41:bool)
  }
  n9 = for {
    tunnel: w8 -> [w46] mode=indexing
    tunnel: [w44] -> w7 mode=indexing
    n10 = Type Cast(type=refnum<k21> "EngineOilPrLamp\nTEST" ("XNET Signal"), x=w46) -> (*(type *) &x=w44:refnum<k21>)
  }
  n11 = for {
    tunnel: w8 -> [w49] mode=indexing
    tunnel: [w48] -> w3 mode=indexing
    tunnel: string[] ["0", "0", "1", "1", "500", "-500", "1", "0", "17000", "300", "-17000", "-300", "0", "1", "0", "500", "500"] ("Array 2") -> [w47] mode=indexing
    n12 = Bundle By Name(cluster=T1 {"FUNCTION"="", "DATA"=""} ("FUNCTIONS"), "FUNCTION"=w49, "DATA"=w47) -> (w48:T1)
  }
  n13 = call "READ CAN DATA.vi"("Enum"=READ_CAN_DATA."SET", "error in (no error)"=w5, "CAN DATA"=w30) -> ("error out"=w6:errorcluster)  [unwired: 7 in, 1 out]
  n14 = call "WRITE EOL TESTFLAG FGV.vi"("Enum"=FGV_States."OPEN", "error in (no error)"=w6, "signal list"=refnum<k21>[] ["Eol_TestFlag\nEDriveMfile_20230607", "MtrInitAngle_CaliFlag\nEDriveMfile_20230607"]) -> ("error out"=w23:errorcluster)  [unwired: 8 in]
  n15 = call "READ FGV.vi"("Enum"=FGV_States."OPEN", "error in (no error)"=w23) -> ("error out"=w22:errorcluster)  [unwired: 8 in, 1 out]
  n16 = property on="WRITE DATA" class="Arr (strict)"("Value"=w3) -> ()  [unwired: 2 in, 2 out]
  n17 = call "WRITE CAN DATA.vi"("Enum"=READ_CAN_DATA."SET", "CAN DATA"=w3) -> ()  [unwired: 9 in, 1 out]
  n18 = call "WRITE FGV.vi"("Enum"=FGV_States."OPEN", "error in (no error)"=w22, "signal list"=w7) -> ("error out"=w24:errorcluster)  [unwired: 8 in]
  n19 = call "Stall Data Flow.vim"("value in"=w24, "milliseconds to wait"=u32 200) -> ("value out"=w10:errorcluster)  [unwired: 1 out]
  n20 = call "WRITE EOL TESTFLAG FGV.vi"("Enum"=FGV_States."WRITE", "error in (no error)"=w10, "data"=dbl[] [1.0, 0.0], "signal list"=refnum<k21>[] ["Eol_TestFlag\nEDriveMfile_20230607", "MtrInitAngle_CaliFlag\nEDriveMfile_20230607"]) -> ("error out"=w26:errorcluster)  [unwired: 7 in]
  n21 = call "Stall Data Flow.vim"("value in"=w26, "milliseconds to wait"=u32 500) -> ("value out"=w27:errorcluster)  [unwired: 1 out]
  n22 = for {
    tunnel: w3 -> [w57] mode=indexing
    tunnel: [w55] -> w25 mode=indexing
    tunnel: refnum<k21> "EngineOilPrLamp\nTEST" ("XNET Signal") -> [w54]
    tunnel: [w52] -> _ mode=indexing
    tunnel: [w51] -> w13
    tunnel: w27 -> [w51]
    n23 = Unbundle By Name(w57) -> ("FUNCTION"=w53:string, "DATA"=w56:string)
    n24 = Type Cast(type=w54, x=w53) -> (*(type *) &x=w52:refnum<k21>)
    n25 = Fract/Exp String To Number(string=w56) -> (number=w55:dbl)  [unwired: 3 in, 1 out]
  }
  n26 = call "WRITE FGV.vi"("Enum"=FGV_States."WRITE", "error in (no error)"=w13, "data"=w25) -> ("error out"=w4:errorcluster)  [unwired: 8 in]
  n27 = while {
    tunnel: w4 -> [w58]
    stop <- "stop" stop-if-true
    n28 = Wait (ms)(milliseconds to wait=u32 100) -> ()  [unwired: 1 out]
    n29 = for {
      tunnel: "WRITE DATA" -> [w84] mode=indexing
      tunnel: [w82] -> w60 mode=indexing
      n30 = Unbundle By Name(w84) -> ("DATA"=w83:string)
      n31 = Fract/Exp String To Number(string=w83) -> (number=w82:dbl)  [unwired: 3 in, 1 out]
    }
    n32 = Or(x="START WRITING", y="Write") -> (x .or. y?=w67:bool)
    n33 = call "READ FGV.vi"("Enum"=FGV_States."READ", "error in (no error)"=w58) -> ("error out"=w69:errorcluster, "data"=w65:dbl[])  [unwired: 8 in]
    n34 = Unbundle By Name(w69) -> ("source"=w77:string, "status"=w78:bool)
    n35 = case shown="True" w67 {
      tunnel: w69 -> [w85 w88]
      tunnel: [w85 w87] -> w63
      tunnel: w60 -> [_ w86]
      frame False {
      }
      frame True {
        n36 = call "WRITE FGV.vi"("Enum"=FGV_States."WRITE", "error in (no error)"=w88, "data"=w86) -> ("error out"=w87:errorcluster)  [unwired: 8 in]
      }
    }
    n37 = call "Read DBC Functions FGV.vi"("Enum"=Read_File_Data."Get Data") -> ("DBC FUNCTIONS OUT"=w74:string[])  [unwired: 9 in, 1 out]
    n38 = Number To Fractional String(number=w65, precision (6)=i16 3) -> (F-format string=w79:string[])  [unwired: 2 in]
    n39 = Select(t=w77, s=w78, f="READING CAN DATA") -> (s? t:f=→"MESSAGES":string)
    n40 = for {
      tunnel: w79 -> [w91] mode=indexing
      tunnel: [w92] -> w72 mode=indexing
      tunnel: w74 -> [w90] mode=indexing
      n41 = Bundle By Name(cluster=T1 {"FUNCTION"="", "DATA"=""} ("FUNCTIONS"), "FUNCTION"=w90, "DATA"=w91) -> (w92:T1)
    }
    "READ DATA" <- w72
    n42 = call "READ CAN DATA.vi"("Enum"=READ_CAN_DATA."SET", "error in (no error)"=w63, "CAN DATA"=w72) -> ("error out"=w61:errorcluster)  [unwired: 7 in, 1 out]
    n43 = call "WRITE CAN DATA DBL.vi"("Enum"=READ_CAN_DATA."SET", "error in (no error)"=w61, "CAN DATA IN"=w60) -> ()  [unwired: 7 in, 2 out]
  }
